vi "While主程序.vi"() -> ()   [LabVIEW 2016]
panel:
  out "输出":dbl
  in  "输入":dbl
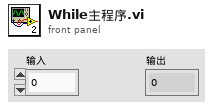
[diagram p1: front panel]
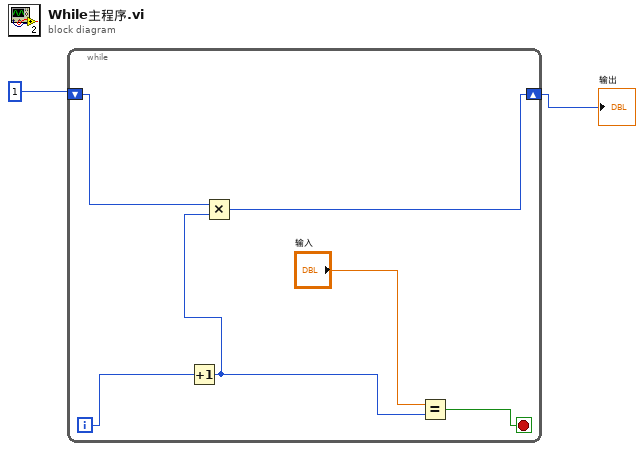
[diagram p0: block diagram]
diagram:
  n1 = while {
    shift-right: [w6] -> w1
    shift-left: 1 -> [w7]
    i -> [w8]
    stop <- w3 stop-if-true
    n2 = Increment(x=w8) -> (x+1=w4:i32)
    n3 = Multiply(x=w7, y=w4) -> (x*y=w6:i32)
    n4 = Equal?(x="输入", y=w4) -> (x = y?=w3:bool)
  }
  "输出" <- w1
